vi "Read Queue and DVR test.vi"() -> ()   [LabVIEW 2021]
uses:
  Master CR.lvclass
  Master CR.lvclass/Master CR.ctl
  Status/Run/Write Run.vi
  Status/write/Write write.vi
  Status/stop/Write stop.vi
  <vilib>/Utility/error.llb/Clear Errors.vi
panel:
  out "x-y 2":u32
  out "x-y":u32
  out "error out":errorcluster
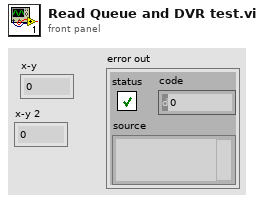
[diagram p1: front panel]
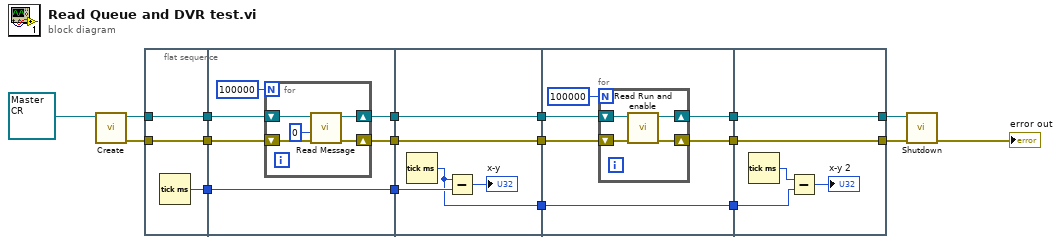
[diagram p0: block diagram]
diagram:
  n1 = call-dynamic "Create.vi"("MB in"=refnum<class "Master CR.lvclass"> refnum ("Master CR in")) -> ("error out"=w17:errorcluster, "MB out"=w16:refnum<class "Master CR.lvclass">)  [unwired: 9 in]
  n2 = flat-sequence {
    tunnel: w16 -> [w20]
    tunnel: w17 -> [w21]
    tunnel: [w21] -> w14
    tunnel: [w20] -> w13
    tunnel: [w19] -> w9
    tunnel: w14 -> [w27]
    tunnel: w13 -> [w26]
    tunnel: [w25] -> w12
    tunnel: [w24] -> w11
    tunnel: [w22] -> w10
    tunnel: w9 -> [w22]
    tunnel: w12 -> [w37]
    tunnel: w11 -> [w36]
    tunnel: w10 -> [w35]
    tunnel: [w37] -> w8
    tunnel: [w36] -> w7
    tunnel: [w33] -> w4
    tunnel: w8 -> [w42]
    tunnel: w7 -> [w43]
    tunnel: w4 -> [w38]
    tunnel: [w41] -> w3
    tunnel: [w40] -> w2
    tunnel: [w38] -> w1
    tunnel: [w51] -> w5
    tunnel: [w52] -> w6
    tunnel: w3 -> [w52]
    tunnel: w2 -> [w51]
    tunnel: w1 -> [w48]
    frame #0 {
      n3 = Tick Count (ms)() -> (millisecond timer value=w19:u32)
    }
    frame #1 {
      n4 = for {
        N: 100000 -> [_]
        shift-right: [w28] -> w24
        shift-left: w27 -> [w32]
        shift-right: [w29] -> w25
        shift-left: w26 -> [w31]
        n5 = call "Read Message.vi"("error in (no error)"=w32, "timeout (0)"=0, "Master CR in"=w31) -> ("error out"=w28:errorcluster, "Master CR out"=w29:refnum<class "Master CR.lvclass">)  [unwired: 6 in, 1 out]
      }
    }
    frame #2 {
      n6 = Tick Count (ms)() -> (millisecond timer value=w33:u32)
      n7 = Subtract(x=w33, y=w35) -> (x-y=→"x-y":u32)
    }
    frame #3 {
      n8 = for {
        N: 100000 -> [_]
        shift-right: [w45] -> w41
        shift-left: w43 -> [w47]
        shift-right: [w44] -> w40
        shift-left: w42 -> [w46]
        n9 = call "Read Run and enable.vi"("error in (no error)"=w47, "Master CR in"=w46) -> ("error out"=w45:errorcluster, "Master CR out"=w44:refnum<class "Master CR.lvclass">)  [unwired: 7 in, 1 out]
      }
    }
    frame #4 {
      n10 = Tick Count (ms)() -> (millisecond timer value=w50:u32)
      n11 = Subtract(x=w50, y=w48) -> (x-y=→"x-y 2":u32)
    }
  }
  n12 = call-dynamic "Shutdown.vi"("error in (no error)"=w6, "MB in"=w5) -> ("error out"=→"error out":errorcluster)  [unwired: 9 in]
